vi "Paths.vi"() -> (3 "Paths":T1)   [LabVIEW 2020, in "FlexBlocks.lvlib"]
uses:
  FlexBlocks.lvlib
  Paths.ctl
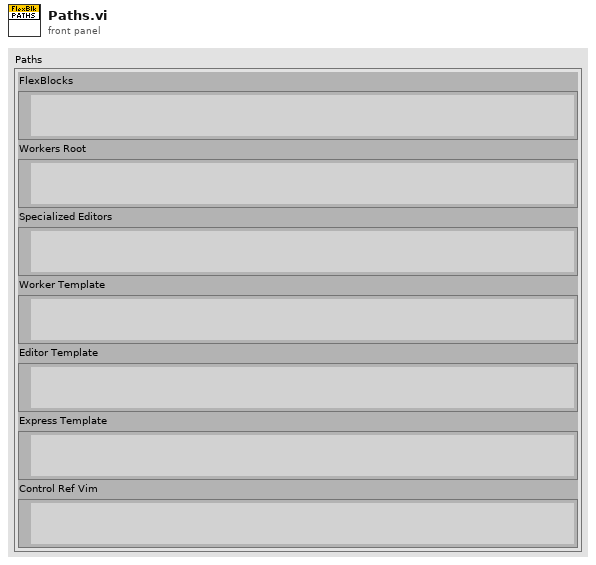
[diagram p1: front panel]
types:
  T1 = typedef "FlexBlocks.lvlib/Paths.ctl" = cluster{"FlexBlocks":path, "Workers Root":path, "Specialized Editors":path, "Worker Template":path, "Editor Template":path, "Express Template":path, "Control Ref Vim":path}
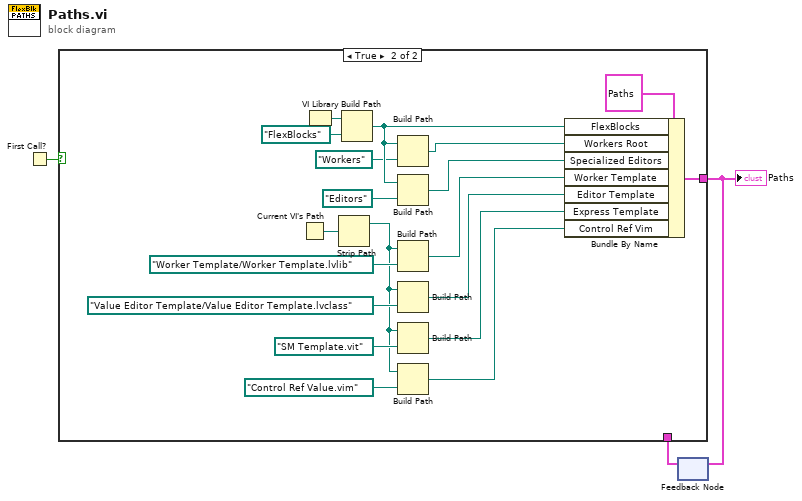
[diagram p0: block diagram]
diagram:
  n1 = First Call?() -> (First Call?: T/F=w3:bool)
  n2 = feedback #1() -> (w1:T1)  [unwired: 1 in]
  n3 = case shown="True" w3 {
    tunnel: [w4 w15] -> w2
    tunnel: w1 -> [w4 _]
    frame False {
    }
    frame True {
      n4 = Current VI's Path() -> (path=w14:path)
      n5 = VI Library() -> (path=w23:path)
      n6 = Strip Path(path=w14) -> (stripped path=w6:path)  [unwired: 1 out]
      n7 = Build Path(base path=w23, name or relative path=path "FlexBlocks") -> (appended path=w20:path)
      n8 = Build Path(base path=w20, name or relative path=path "Workers") -> (appended path=w18:path)
      n9 = Build Path(base path=w20, name or relative path=path "Editors") -> (appended path=w16:path)
      n10 = Build Path(base path=w6, name or relative path=path "Worker Template/Worker Template.lvlib") -> (appended path=w10:path)
      n11 = Build Path(base path=w6, name or relative path=path "Value Editor Template/Value Editor Template.lvclass") -> (appended path=w9:path)
      n12 = Build Path(base path=w6, name or relative path=path "SM Template.vit") -> (appended path=w8:path)
      n13 = Build Path(base path=w6, name or relative path=path "Control Ref Value.vim") -> (appended path=w5:path)
      n14 = Bundle By Name(cluster=T1 {"FlexBlocks"=path "", "Workers Root"=path "", "Specialized Editors"=path "", "Worker Template"=path "", "Editor Template"=path "", "Express Template"=path "", "Control Ref Vim"=path ""} ("Paths"), "FlexBlocks"=w20, "Workers Root"=w18, "Specialized Editors"=w16, "Worker Template"=w10, "Editor Template"=w9, "Express Template"=w8, "Control Ref Vim"=w5) -> (w15:T1)
    }
  }
  "Paths" <- w2
  n15 = feedback-in #1(w2) -> ()
